vi "EditValueCore.vi"(8 "error in (no error)":errorcluster, 9 "Value field reference":refnum<vi>, 10 "Bounds":T1, 11 "DatagridElement in":refnum<class "DatagridElement.lvclass">) -> (0 "error out":errorcluster, 1 "Tabbed out?":bool, 2 "Value changed?":bool, 3 "DatagridElement out":refnum<class "DatagridElement.lvclass">)   [LabVIEW 2018, in "D Datagrid Library.lvlib" / "DatagridElement.lvclass"]
uses:
  DatagridElement.lvclass
  <vilib>/Utility/miscctls.llb/LVRectTypeDef.ctl
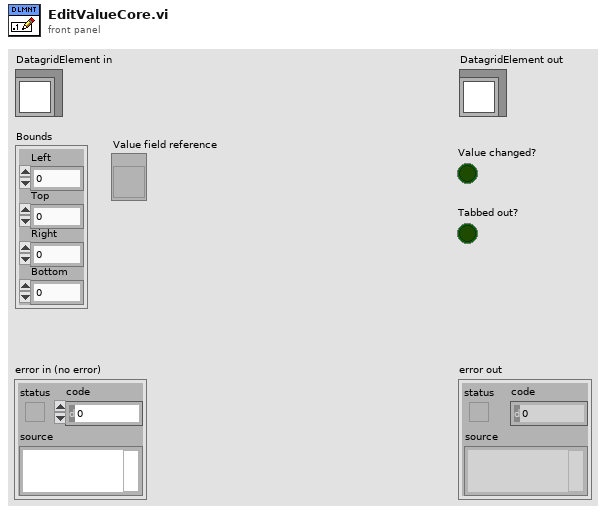
[diagram p1: front panel]
types:
  T1 = typedef "LVRectTypeDef.ctl" = cluster{"Left":i16, "Top":i16, "Right":i16, "Bottom":i16}
  T2 = enum32{"Invalid", "Standard", "Closed", "Hidden", "Minimized", "Maximized"}
  T3 = enum32{"Invalid", "Default", "Floating", "Floating/Auto-Hide", "Modal"}
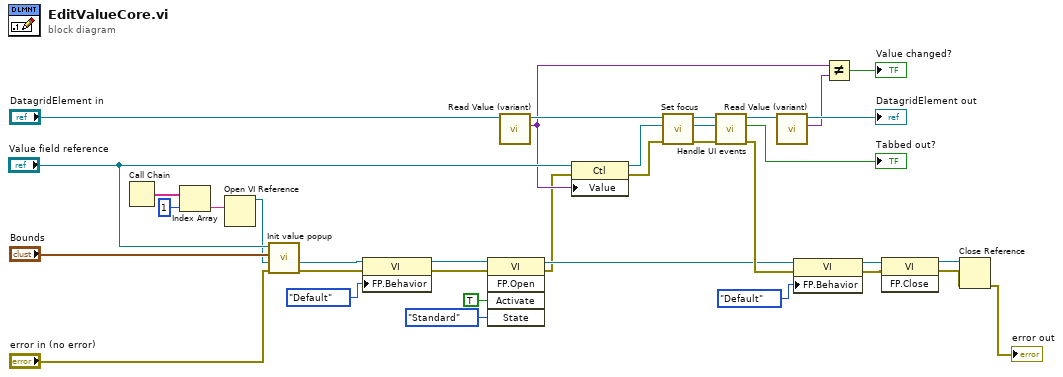
[diagram p0: block diagram]
diagram:
  n1 = Call Chain() -> (call chain=w31:string[])
  n2 = Index Array(array=w31, index=1) -> (element=w29:string)
  n3 = Open VI Reference(vi path=w29) -> (vi reference=w16:refnum<vi>)  [unwired: 5 in, 1 out]
  n4 = call "Init value popup.vi"("error in (no error)"="error in (no error)", "Popup window reference"=w16, "Bounds"="Bounds", "Control reference size override (none)"="Value field reference") -> ("error out"=w15:errorcluster, "Popup window reference out"=w6:refnum<vi>)  [unwired: 6 in]
  n5 = property class="VI"(reference=w6, error in=w15, "FP.Behavior"=T3."Default" ("Front Panel Window:Behavior")) -> (reference out=w7:refnum<vi>, error out=w8:errorcluster)
  n6 = invoke class="VI" method="FP.Open"(reference=w7, error in=w8, "Activate"=TRUE ("Activate?"), "State"=T2."Standard") -> (reference out=w11:refnum<vi>, error out=w9:errorcluster)  [unwired: 1 in, 3 out]
  n7 = call-dynamic "Read Value (variant).vi"("DatagridElement in"="DatagridElement in") -> ("Variant"=w20:variant, "DatagridElement out"=w26:refnum<class "DatagridElement.lvclass">)  [unwired: 8 in, 1 out]
  n8 = property class="Ctl"(reference="Value field reference", error in=w9, "Value"=w20) -> (reference out=w28:refnum<vi>, error out=w27:errorcluster)
  n9 = call-dynamic "Set focus.vi"("error in (no error)"=w27, "Control ref"=w28, "DatagridElement in"=w26) -> ("error out"=w24:errorcluster, "Control out"=w18:refnum<vi>, "DatagridElement out"=w25:refnum<class "DatagridElement.lvclass">)  [unwired: 6 in]
  n10 = call-dynamic "Handle UI events.vi"("error in (no error)"=w24, "Control in"=w18, "DatagridElement in"=w25) -> ("error out"=w12:errorcluster, "Tabbed out?"=→"Tabbed out?":bool, "DatagridElement out"=w23:refnum<class "DatagridElement.lvclass">)  [unwired: 6 in]
  n11 = call-dynamic "Read Value (variant).vi"("DatagridElement in"=w23) -> ("Variant"=w21:variant, "DatagridElement out"=→"DatagridElement out":refnum<class "DatagridElement.lvclass">)  [unwired: 8 in, 1 out]
  n12 = property class="VI"(reference=w11, error in=w12, "FP.Behavior"=T3."Default" ("Front Panel Window:Behavior")) -> (reference out=w13:refnum<vi>, error out=w5:errorcluster)
  n13 = Not Equal?(x=w20, y=w21) -> (x != y?=→"Value changed?":bool)
  n14 = invoke class="VI" method="FP.Close"(reference=w13, error in=w5) -> (reference out=w35:refnum<vi>, error out=w4:errorcluster)  [unwired: 1 in, 1 out]
  n15 = Close Reference(reference=w35, error in (no error)=w4) -> (error out=→"error out":errorcluster)
